vi "main.vi"() -> ()   [LabVIEW 2014]
uses:
  vi.lib/Q-WaveSystems/QwaveSys Raspberry Pi for LabVIEW Home-Education/WiringPi/WiringPi GPIO TypeDef.ctl
  vi.lib/Q-WaveSystems/QwaveSys Raspberry Pi for LabVIEW Home-Education/WiringPi/WiringPi Pin Mode.ctl
  led.vi
  led2.vi
  led3.vi
  led4.vi
  counter.vi
  vi.lib/Q-WaveSystems/QwaveSys Raspberry Pi for LabVIEW Home-Education/QwaveSys Raspberry Pi Library.lvlib
panel:
  in  "WiringPi GPIO 4":T1=7 items=["SDA(I2C)-3"=8, "SCL(I2C)-5"=9, "MOSI(SPI)-19"=12, "MISO(SPI)-21"=13, "SCLK(SPI)-23"=14, "GPIO2-13"=2, "GPIO3-15"=3, "GPIO4-16"=4, "GPIO5-18"=5, "GPIO6-22"=6, "GPIO7-7"=7, "GPIO21-29"=21, "GPIO22-31"=22, "GPIO25-37"=25, "GPIO27-36"=27, "GPIO26(PWM0)-32"=26, "GPIO1(PWM0-12)"=1, "GPIO23(PWM1)-14"=23, "GPIO24(PWM1)-35"=24, "TXD(UART)-8"=15, "RXD(UART)-10"=16, "GPIO10(CE0-SPI)-24"=10, "GPPI11(CE1)-SPI)-26"=11, "GPIO28(PCM_DIN)36"=28, "GPIO29(PCM_DOUT)40"=29]
  in  "WiringPi GPIO 3":T1=7 items=["SDA(I2C)-3"=8, "SCL(I2C)-5"=9, "MOSI(SPI)-19"=12, "MISO(SPI)-21"=13, "SCLK(SPI)-23"=14, "GPIO2-13"=2, "GPIO3-15"=3, "GPIO4-16"=4, "GPIO5-18"=5, "GPIO6-22"=6, "GPIO7-7"=7, "GPIO21-29"=21, "GPIO22-31"=22, "GPIO25-37"=25, "GPIO27-36"=27, "GPIO26(PWM0)-32"=26, "GPIO1(PWM0-12)"=1, "GPIO23(PWM1)-14"=23, "GPIO24(PWM1)-35"=24, "TXD(UART)-8"=15, "RXD(UART)-10"=16, "GPIO10(CE0-SPI)-24"=10, "GPPI11(CE1)-SPI)-26"=11, "GPIO28(PCM_DIN)36"=28, "GPIO29(PCM_DOUT)40"=29]
  in  "WiringPi GPIO 2":T1=7 items=["SDA(I2C)-3"=8, "SCL(I2C)-5"=9, "MOSI(SPI)-19"=12, "MISO(SPI)-21"=13, "SCLK(SPI)-23"=14, "GPIO2-13"=2, "GPIO3-15"=3, "GPIO4-16"=4, "GPIO5-18"=5, "GPIO6-22"=6, "GPIO7-7"=7, "GPIO21-29"=21, "GPIO22-31"=22, "GPIO25-37"=25, "GPIO27-36"=27, "GPIO26(PWM0)-32"=26, "GPIO1(PWM0-12)"=1, "GPIO23(PWM1)-14"=23, "GPIO24(PWM1)-35"=24, "TXD(UART)-8"=15, "RXD(UART)-10"=16, "GPIO10(CE0-SPI)-24"=10, "GPPI11(CE1)-SPI)-26"=11, "GPIO28(PCM_DIN)36"=28, "GPIO29(PCM_DOUT)40"=29]
  in  "WiringPi GPIO":T1=7 items=["SDA(I2C)-3"=8, "SCL(I2C)-5"=9, "MOSI(SPI)-19"=12, "MISO(SPI)-21"=13, "SCLK(SPI)-23"=14, "GPIO2-13"=2, "GPIO3-15"=3, "GPIO4-16"=4, "GPIO5-18"=5, "GPIO6-22"=6, "GPIO7-7"=7, "GPIO21-29"=21, "GPIO22-31"=22, "GPIO25-37"=25, "GPIO27-36"=27, "GPIO26(PWM0)-32"=26, "GPIO1(PWM0-12)"=1, "GPIO23(PWM1)-14"=23, "GPIO24(PWM1)-35"=24, "TXD(UART)-8"=15, "RXD(UART)-10"=16, "GPIO10(CE0-SPI)-24"=10, "GPPI11(CE1)-SPI)-26"=11, "GPIO28(PCM_DIN)36"=28, "GPIO29(PCM_DOUT)40"=29]
  out "led4":bool
  out "led3":bool
  out "led2":bool
  out "TempC":dbl
  out "led":bool
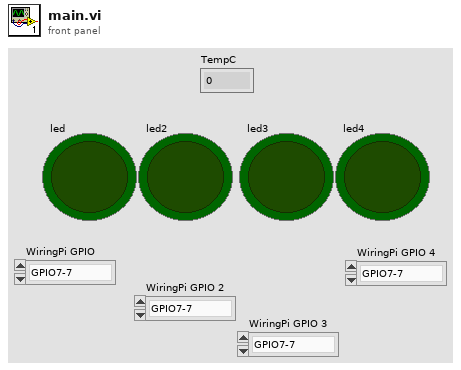
[diagram p1: front panel]
types:
  T1 = typedef "QwaveSys Raspberry Pi Library.lvlib/WiringPi GPIO TypeDef.ctl" = u8
  T2 = typedef "QwaveSys Raspberry Pi Library.lvlib/WiringPi Pin Mode.ctl" = enum8{"INPUT", "OUTPUT", "PWM_OUTPUT", "GPIO_CLOCK", "SOFT_PWM_OUTPUT", "SOFT_TONE_OUTPUT", "PWM_TONE_OUTPUT"}
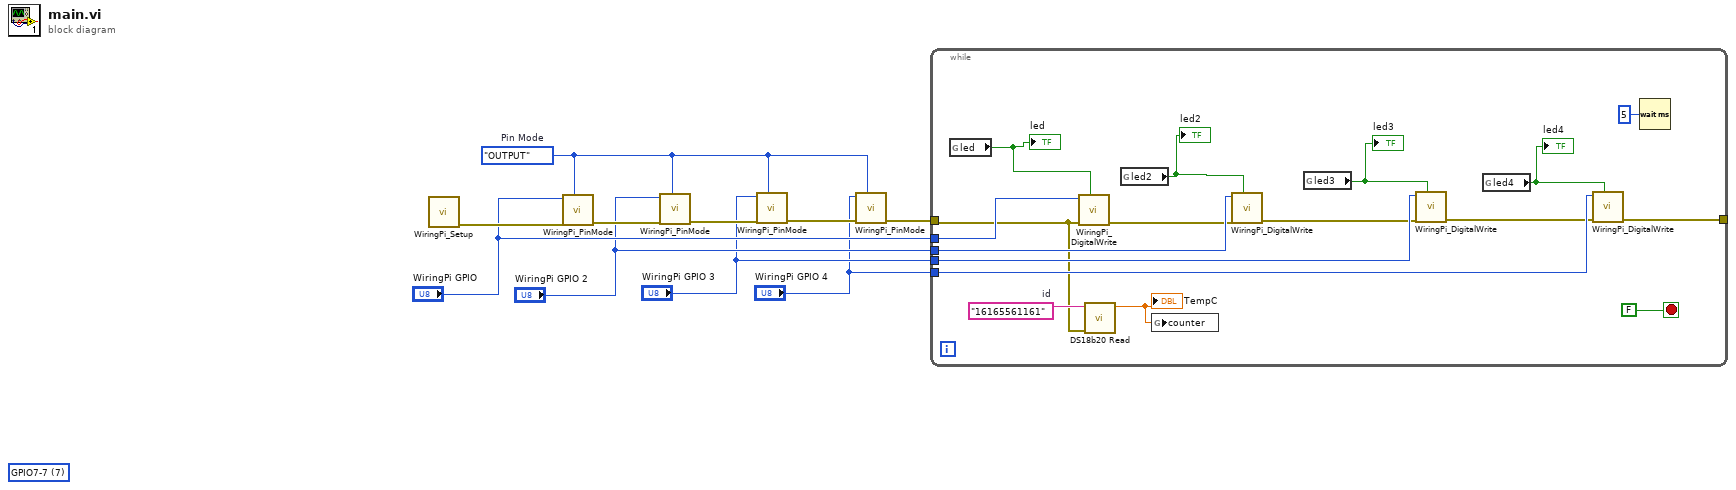
[diagram p0: block diagram]
diagram:
  w6 = WiringPi_Pin_Mode."OUTPUT"  # Pin Mode
  (unwired) u8 7 items=["SDA(I2C)-3"=8, "SCL(I2C)-5"=9, "MOSI(SPI)-19"=12, "MISO(SPI)-21"=13, "SCLK(SPI)-23"=14, "GPIO2-13"=2, "GPIO3-15"=3, "GPIO4-16"=4, "GPIO5-18"=5, "GPIO6-22"=6, "GPIO7-7"=7, "GPIO21-29"=21, "GPIO22-31"=22, "GPIO25-37"=25, "GPIO27-36"=27, "GPIO26(PWM0)-32"=26, "GPIO1(PWM0-12)"=1, "GPIO23(PWM1)-14"=23, "GPIO24(PWM1)-35"=24, "TXD(UART)-8"=15, "RXD(UART)-10"=16, "GPIO10(CE0-SPI)-24"=10, "GPPI11(CE1)-SPI)-26"=11, "GPIO28(PCM_DIN)36"=28, "GPIO29(PCM_DOUT)40"=29] ("WiringPi GPIO")
  n1 = call "WiringPi_Setup.vi"() -> ("error out"=w10:errorcluster)  [unwired: 11 in]
  n2 = call "WiringPi_PinMode.vi"("Pin Mode"=w6, "error in (no error)"=w10, "WiringPi GPIO"="WiringPi GPIO") -> ("error out"=w9:errorcluster)  [unwired: 8 in]
  n3 = call "WiringPi_PinMode.vi"("Pin Mode"=w6, "error in (no error)"=w9, "WiringPi GPIO"="WiringPi GPIO 2") -> ("error out"=w8:errorcluster)  [unwired: 8 in]
  n4 = call "WiringPi_PinMode.vi"("Pin Mode"=w6, "error in (no error)"=w8, "WiringPi GPIO"="WiringPi GPIO 3") -> ("error out"=w7:errorcluster)  [unwired: 8 in]
  n5 = call "WiringPi_PinMode.vi"("Pin Mode"=w6, "error in (no error)"=w7, "WiringPi GPIO"="WiringPi GPIO 4") -> ("error out"=w5:errorcluster)  [unwired: 8 in]
  n6 = while {
    tunnel: w5 -> [w15]
    tunnel: "WiringPi GPIO" -> [w25]
    tunnel: "WiringPi GPIO 2" -> [w24]
    tunnel: "WiringPi GPIO 3" -> [w23]
    tunnel: "WiringPi GPIO 4" -> [w22]
    tunnel: [w18] -> _
    stop <- FALSE stop-if-true
    w17 = "16165561161"  # id
    n7 = global read "led.vi" "led"() -> (w14:bool)
    "led" <- w14
    n8 = call "WiringPi_DigitalWrite.vi"("Value"=w14, "error in (no error)"=w15, "WiringPi GPIO"=w25) -> ("error out"=w21:errorcluster)  [unwired: 8 in]
    n9 = call "DS18b20 Read.vi"("error in (no error)"=w15, "id"=w17) -> ("Temp"=w16:dbl)  [unwired: 8 in, 1 out]
    "TempC" <- w16
    n10 = global read "led2.vi" "led2"() -> (w13:bool)
    "led2" <- w13
    n11 = global write "counter.vi" "counter"(w16) -> ()
    n12 = call "WiringPi_DigitalWrite.vi"("Value"=w13, "error in (no error)"=w21, "WiringPi GPIO"=w24) -> ("error out"=w20:errorcluster)  [unwired: 8 in]
    n13 = global read "led3.vi" "led3"() -> (w12:bool)
    "led3" <- w12
    n14 = call "WiringPi_DigitalWrite.vi"("Value"=w12, "error in (no error)"=w20, "WiringPi GPIO"=w23) -> ("error out"=w19:errorcluster)  [unwired: 8 in]
    n15 = global read "led4.vi" "led4"() -> (w11:bool)
    "led4" <- w11
    n16 = call "WiringPi_DigitalWrite.vi"("Value"=w11, "error in (no error)"=w19, "WiringPi GPIO"=w22) -> ("error out"=w18:errorcluster)  [unwired: 8 in]
    n17 = Wait (ms)(milliseconds to wait=u32 5) -> ()  [unwired: 1 out]
  }
